vi "Send Pulse.vi"(8 "error in (no error)":errorcluster, 11 "Sync Box in":refnum<class "Sync Box.lvclass">) -> (0 "error out":errorcluster, 3 "Sync Box out":refnum<class "Sync Box.lvclass">)   [LabVIEW 2018, in "Sync Box.lvclass"]
uses:
  Sync Box.lvclass
  Sync Box.lvclass/Sync Box.ctl
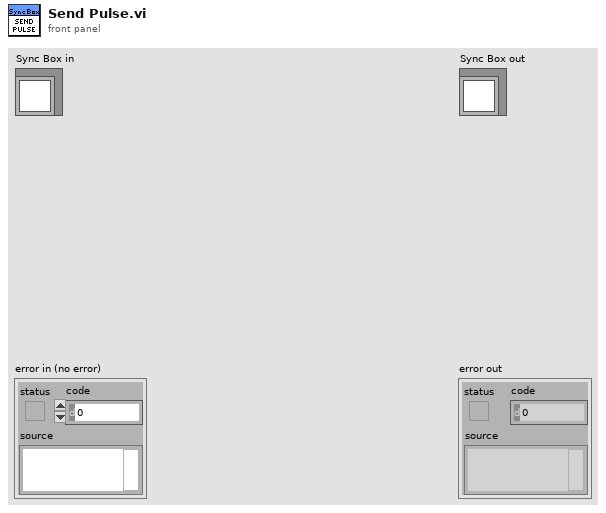
[diagram p1: front panel]
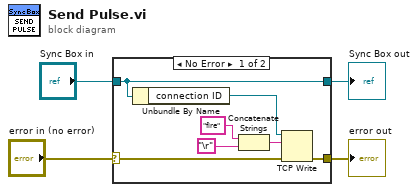
[diagram p0: block diagram]
diagram:
  n1 = case shown="No Error" "error in (no error)" {
    selector: "error in (no error)" -> [w11 w13]
    tunnel: [w10 w13] -> w3
    tunnel: [w5 w12] -> w1
    tunnel: "Sync Box in" -> [w5 w12]
    frame No Error {
      n2 = Unbundle By Name(w5) -> ("connection ID"=w9:refnum<k5>)
      n3 = Concatenate Strings("fire", "\r") -> (w8:string)
      n4 = TCP Write(connection ID=w9, data in=w8, error in (no error)=w11) -> (error out=w10:errorcluster)  [unwired: 1 in, 2 out]
    }
    frame Error {
    }
  }
  "error out" <- w3
  "Sync Box out" <- w1
